vi "Find_Row_Shaft_in.vi"(0 "Basic Size":ext, 5 "error in (no error)":errorcluster) -> (6 "Row":ext, 8 "error out":errorcluster)   [LabVIEW 2023]
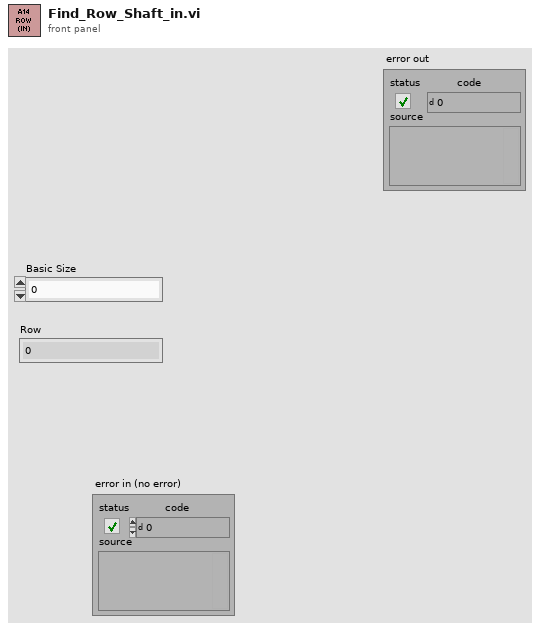
[diagram p1: front panel]
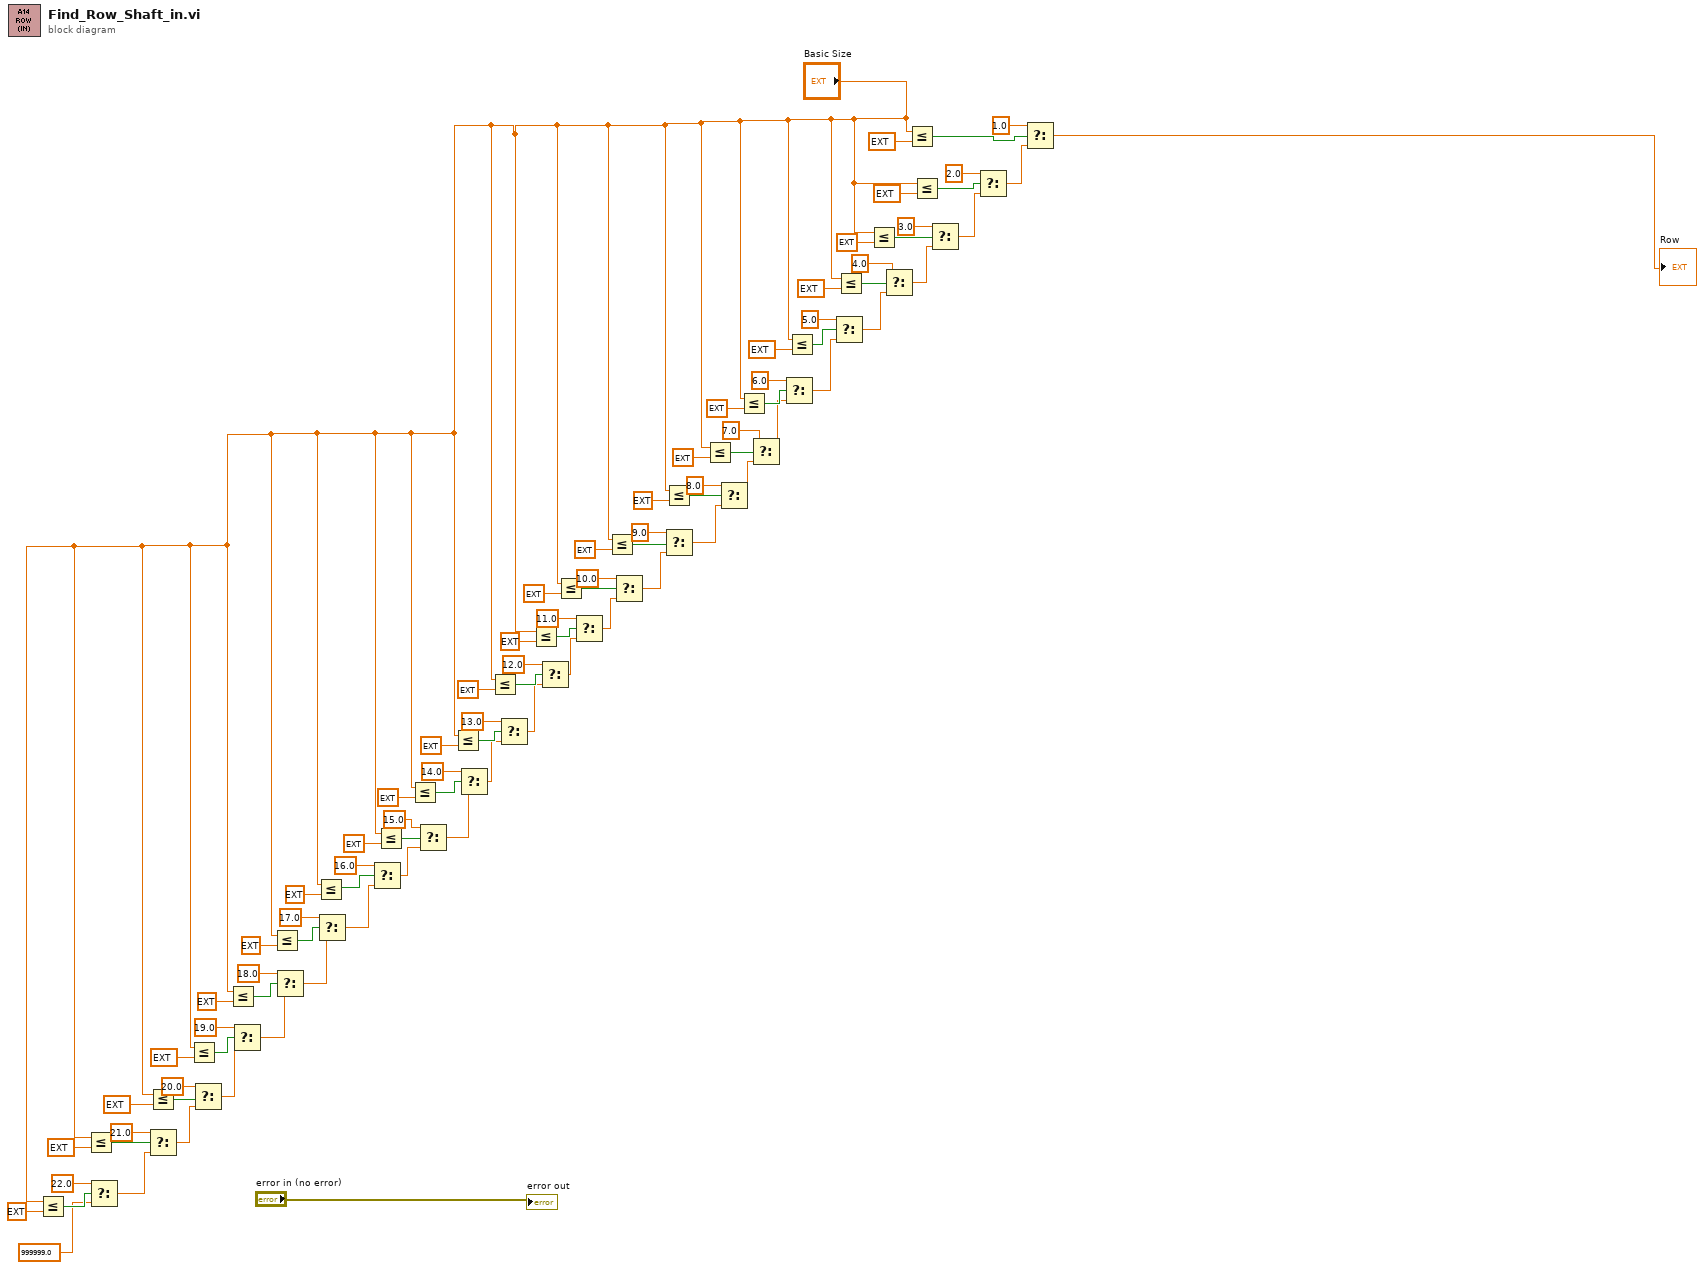
[diagram p0: block diagram]
diagram:
  n1 = Less Or Equal?(x="Basic Size", y=ext 16.0) -> (x <= y?=w5:bool)
  n2 = Less Or Equal?(x="Basic Size", y=ext 14.2) -> (x <= y?=w9:bool)
  n3 = Select(t=22.0, s=w5, f=999999.0) -> (s? t:f=w7:dbl)
  n4 = Less Or Equal?(x="Basic Size", y=ext 12.6000000000000000003) -> (x <= y?=w14:bool)
  n5 = Select(t=21.0, s=w9, f=w7) -> (s? t:f=w12:dbl)
  n6 = Less Or Equal?(x="Basic Size", y=ext 11.2) -> (x <= y?=w17:bool)
  n7 = Select(t=20.0, s=w14, f=w12) -> (s? t:f=w15:dbl)
  n8 = Less Or Equal?(x="Basic Size", y=ext 10.0) -> (x <= y?=w21:bool)
  n9 = Select(t=19.0, s=w17, f=w15) -> (s? t:f=w19:dbl)
  n10 = Less Or Equal?(x="Basic Size", y=ext 9.0) -> (x <= y?=w25:bool)
  n11 = Select(t=18.0, s=w21, f=w19) -> (s? t:f=w23:dbl)
  n12 = Less Or Equal?(x="Basic Size", y=ext 8.0) -> (x <= y?=w29:bool)
  n13 = Select(t=17.0, s=w25, f=w23) -> (s? t:f=w27:dbl)
  n14 = Select(t=16.0, s=w29, f=w27) -> (s? t:f=w31:dbl)
  n15 = Less Or Equal?(x="Basic Size", y=ext 7.2) -> (x <= y?=w33:bool)
  n16 = Less Or Equal?(x="Basic Size", y=ext 6.4) -> (x <= y?=w37:bool)
  n17 = Select(t=15.0, s=w33, f=w31) -> (s? t:f=w35:dbl)
  n18 = Less Or Equal?(x="Basic Size", y=ext 5.6) -> (x <= y?=w41:bool)
  n19 = Select(t=14.0, s=w37, f=w35) -> (s? t:f=w39:dbl)
  n20 = Less Or Equal?(x="Basic Size", y=ext 4.8000000000000000002) -> (x <= y?=w45:bool)
  n21 = Select(t=13.0, s=w41, f=w39) -> (s? t:f=w43:dbl)
  n22 = Less Or Equal?(x="Basic Size", y=ext 4.0) -> (x <= y?=w49:bool)
  n23 = Select(t=12.0, s=w45, f=w43) -> (s? t:f=w47:dbl)
  n24 = Less Or Equal?(x="Basic Size", y=ext 3.2) -> (x <= y?=w53:bool)
  n25 = Select(t=11.0, s=w49, f=w47) -> (s? t:f=w51:dbl)
  n26 = Less Or Equal?(x="Basic Size", y=ext 2.5999999999999999999) -> (x <= y?=w57:bool)
  n27 = Select(t=10.0, s=w53, f=w51) -> (s? t:f=w55:dbl)
  n28 = Less Or Equal?(x="Basic Size", y=ext 2.0) -> (x <= y?=w61:bool)
  n29 = Select(t=9.0, s=w57, f=w55) -> (s? t:f=w59:dbl)
  n30 = Less Or Equal?(x="Basic Size", y=ext 1.6) -> (x <= y?=w65:bool)
  n31 = Select(t=8.0, s=w61, f=w59) -> (s? t:f=w63:dbl)
  n32 = Less Or Equal?(x="Basic Size", y=ext 1.20000000000000000004) -> (x <= y?=w69:bool)
  n33 = Select(t=7.0, s=w65, f=w63) -> (s? t:f=w67:dbl)
  n34 = Select(t=6.0, s=w69, f=w67) -> (s? t:f=w71:dbl)
  n35 = Less Or Equal?(x="Basic Size", y=ext 0.96) -> (x <= y?=w73:bool)
  n36 = Select(t=5.0, s=w73, f=w71) -> (s? t:f=w75:dbl)
  n37 = Less Or Equal?(x="Basic Size", y=ext 0.72000000000000000003) -> (x <= y?=w78:bool)
  n38 = Less Or Equal?(x="Basic Size", y=ext 0.4) -> (x <= y?=w82:bool)
  n39 = Select(t=4.0, s=w78, f=w75) -> (s? t:f=w79:dbl)
  n40 = Less Or Equal?(x="Basic Size", y=ext 0.12) -> (x <= y?=w86:bool)
  n41 = Less Or Equal?(x="Basic Size", y=ext 0.24) -> (x <= y?=w85:bool)
  n42 = Select(t=3.0, s=w82, f=w79) -> (s? t:f=w83:dbl)
  n43 = Select(t=2.0, s=w85, f=w83) -> (s? t:f=w90:dbl)
  n44 = Select(t=1.0, s=w86, f=w90) -> (s? t:f=→"Row":dbl)
  "error out" <- "error in (no error)"
